vi "Josey buffered mod.vi"() -> ()   [LabVIEW 2010]
uses:
  <vilib>/Utility/file.llb/Write To Spreadsheet File (I64).vi
panel:
  out "Peak to Peak":dbl
  in  "Auto Save Data":bool=TRUE
  out "date/time string":string="2012-02-20 12-35.08"
  in  "time format string (%c)":string="%Y-%m-%d %H-%M.%S"
  in  "Data file path ending":string=".dat"
  out "Previous acquisition":u16[](graph)
  in  "LowChan":i32
  in  "HighChan":i32
  in  "Count":i32=1000
  in  "Rate":i32=3000
  in  "Options":i32
  in  "InterChannel Delay":sgl=-1.0 format="%.2f"
  in  "Range":i32(ring)=1 items=["Not Programmable"=0, "+- 20 V"=27, "+- 10 V"=1, "+- 5 V"=2, "+- 4 V"=28, "+- 2.5 V"=3, "+- 2 V"=29, "+- 1.67 V"=4, "+- 1.25 V"=5, "+- 1 V"=6, "+- .625 V"=7, "+- .5 V"=8, "+- .25 V"=30, "+- .2 V"=31, "+- .1 V"=9, "+- .05 V"=10, "+- .01 V"=11, "+- .005 V"=12, "0 - 10 V"=13, "0 - 5 V"=14, "0 - 4 V"=36, "0 - 2.5 V"=15, "0 - 2 V"=16, "0 - 1.67 V"=17, "0 - 1.25 V"=18, "0 - 1 V"=19, "0 - .5 V"=32, "0 - .25 V"=33, "0 - .2 V"=34, "0 - .1 V"=20, "0 - .02 V"=35, "0 - .01 V"=21, "4 - 20 mA"=22, "2 - 10 mA"=23, "1 - 5 mA"=24, ".5 - 2.5 mA"=25, "0 - 20 mA"=26]
  out "Current acquisition":u16[](graph)
  out "ErrCode":i32
  out "ErrMsg":string="No error has occurred"
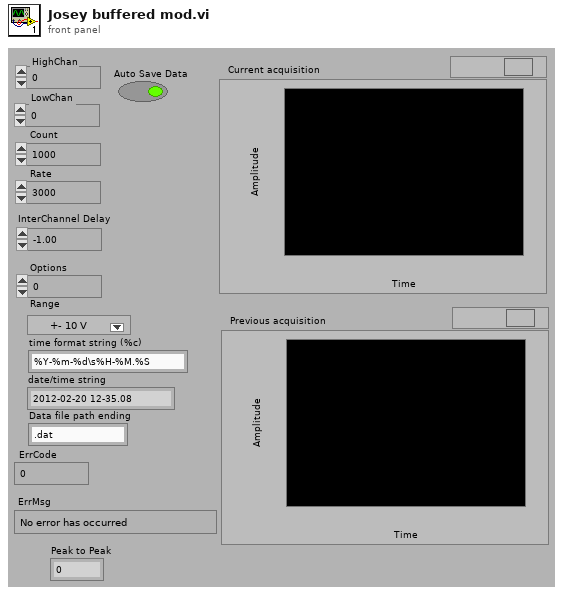
[diagram p1: front panel]
types:
  T1 = typedef "imagedata.ctl" = cluster{"image type":i32, "image depth":i32, "image":u8[], "mask":u8[], "colors":u32[], "Rectangle":cluster{"left":i16, "top":i16, "right":i16, "bottom":i16}}
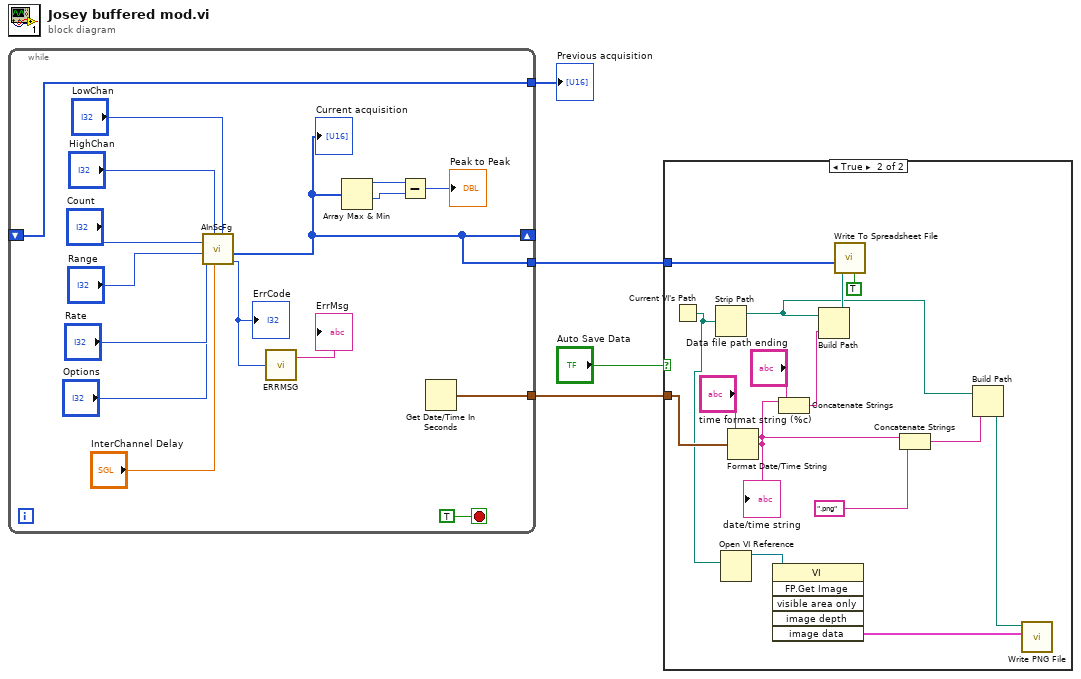
[diagram p0: block diagram]
diagram:
  n1 = while {
    shift-right: [w8] -> _
    shift-left: _ -> [w10]
    tunnel: [w10] -> w4
    tunnel: [w8] -> w3
    tunnel: [w9] -> w2
    stop <- TRUE stop-if-true
    n2 = call <menus>:"AInScFg.VI"("LowChan"="LowChan", "InterChannel Delay"="InterChannel Delay", "HighChan"="HighChan", "Options"="Options", "Range"="Range", "Rate"="Rate", "Count"="Count") -> ("ErrCode"=w13:i32, "ADData"=w8:u16[])  [unwired: 1 in, 1 out]
    "Current acquisition" <- w8
    "ErrCode" <- w13
    n3 = call <menus>:"ERRMSG.VI"("ErrCode"=w13) -> ("ErrMsg"=→"ErrMsg":string)  [unwired: 1 out]
    n4 = Array Max & Min(array=w8) -> (max value=w7:u16, min value=w6:u16)  [unwired: 2 out]
    n5 = Subtract(x=w7, y=w6) -> (x-y=→"Peak to Peak":u16)
    n6 = Get Date/Time In Seconds() -> (seconds since 1Jan1904=w9:timestamp)
  }
  "Previous acquisition" <- w4
  n7 = case shown="True" "Auto Save Data" {
    tunnel: w3 -> [_ w35]
    tunnel: w2 -> [_ w34]
    frame False {
    }
    frame True {
      n8 = Current VI's Path() -> (path=w26:path)
      n9 = Strip Path(path=w26) -> (stripped path=w25:path)  [unwired: 1 out]
      n10 = Open VI Reference(vi path=w26) -> (vi reference=w27:refnum<vi>)  [unwired: 5 in, 1 out]
      n11 = Format Date/Time String(time format string (%c)="time format string (%c)", seconds (now)=w34) -> (date/time string=w24:string)  [unwired: 1 in]
      "date/time string" <- w24
      n12 = invoke class="VI" method="FP.Get Image"(reference=w27) -> ("image data"=w28:T1)  [unwired: 5 in, 5 out]
      n13 = Concatenate Strings(w24, "Data file path ending") -> (w31:string)
      n14 = Build Path(base path=w25, name or relative path=w31) -> (appended path=w30:path)
      n15 = call-poly <vilib>:"Write To Spreadsheet File.vi"("transpose? (no:F)"=TRUE, "1D data"=w35, "file path (dialog if empty)"=w30) -> ()  [unwired: 5 in, 1 out]
      n16 = Concatenate Strings(w24, ".png" ("string")) -> (w22:string)
      n17 = Build Path(base path=w25, name or relative path=w22) -> (appended path=w21:path)
      n18 = call <vilib>:"Write PNG File.vi"("image data"=w28, "path to PNG file"=w21) -> ()  [unwired: 8 in, 2 out]
    }
  }
